vi "CSM - Flush Queue.vi"(8 "Error In":errorcluster caption="error in (no error)", 9 "Option (Low Priority As Default)":enum16{"All", "High Priority", "Low Priority"}(ring)=enum."Low Priority", 11 "CSM Name":string) -> (0 "error out":errorcluster, 1 "#Flushed":cluster{i32, i32}, 3 "CSM Name (Dup)":string)   [LabVIEW 2017, in "Communicable State Machine.lvlib"]
doc: "Clears the LabVIEW queue used in the background for inter-module communication of a CSM module.\n\n> [!NOTE] \n> <b>CSM Priority Queue Design</b>\n>\n> In the background, CSM essentially uses LabVIEW queues to implement inter-module communication. However, CSM uses two separate queues to store messages of different priorities:\n>\n> - <b>Normal Priority Queue:</b> Used for passing asynchronous messages and status broadcasts.\n> - <b>High Priority Message Queue:</b> Used for passing synchronous messages and interrupt broadcasts. Messages in the High Priority Queue are processed first. Messages in the Normal Priority Queue are processed only after the messages in the High Priority Queue have been processed.\n\n\n> [!WARNING] \n> Using this VI is generally not recommended for CSM modules. It is recommended to use code design to avoid message accumulation in modules. Therefore, it is recommended to avoid using this VI to clear background message queues in CSM modules.\n\n-- <b>Controls</b> --\n- <b>CSM Name</b>: CSM module name.\n- <b>Option (Low Priority As Default)</b>: The queue to flush. You can select from the following: All, Low Priority, and High Priority. The default is Low Priority.\n\n-- <b>Indicators</b> --\n- <b>CSM Name (Dup)</b>: A copy of the input CSM module name.\n- <b>#Flushed</b>: Number of elements in the flushed message queue."
uses:
  Communicable State Machine.lvlib
  _Support/CSMQ/_CSMOFGVOPER.ctl
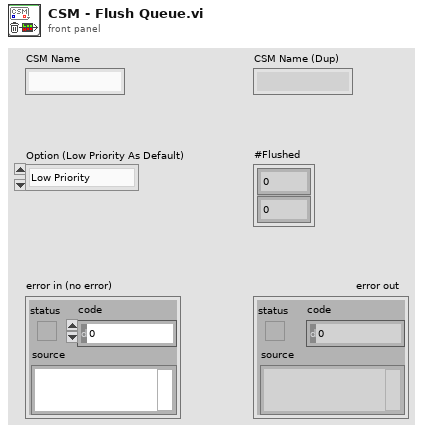
[diagram p1: front panel]
types:
  T1 = typedef "Communicable State Machine.lvlib/_CSMOFGVOPER.ctl" = enum16{"Create If not Exist", "Get By Name", "List", "Check If Name Exists", "Release", "Module Status", "Create Status Event Handler", "Destroy Status Event Handler", "Clear Invalid Objs"}
  T2 = typedef "Communicable State Machine.lvlib/_CSMObj.ctl" = cluster{"info":T3, "Refs":T5}
  T3 = typedef "Communicable State Machine.lvlib/_CSMObj-Info.ctl" = cluster{"Module Name":string, "Requested Name":string, "Group Name":string, "Mode":T4, "Allowed Messages":string[]}
  T4 = typedef "Communicable State Machine.lvlib/_CSM_MODE.ctl" = enum16{"Not Exist", "Stand Alone", "CSM", "Worker", "Worker Agent", "Chain Node", "Chain"}
  T5 = typedef "Communicable State Machine.lvlib/_CSMObj-Refs.ctl" = cluster{"WatchDogQ":refnum<queue>, "CSMDataDVR":refnum<data-value>, "Queue":T6, "GroupDataDVR":refnum<data-value>, "TagMap":refnum<data-value>, "ExitEvent":refnum<user-event>, "NewStateEvent":refnum<user-event>, "StatusEvent":refnum<user-event>, "InterruptEvent":refnum<user-event>}
  T6 = typedef "Communicable State Machine.lvlib/Priority Queue.ctl" = cluster{"HPriorityQ":refnum<queue>, "LowPriorityQ":refnum<queue>}
  T7 = typedef "Communicable State Machine.lvlib/def-Data(LowPRI-Q).ctl" = cluster{"Data":T8, "Notify?":bool}
  T8 = typedef "Communicable State Machine.lvlib/_Cross CSM State Data.ctl" = cluster{"Msg Type":T9, "state":string, "args":string, "source":string, "RespQ":refnum<queue>, "Response For Message":T10, "Target":string}
  T9 = typedef "Communicable State Machine.lvlib/_CSM_MSG_TYPE.ctl" = enum16{"Sync Message(-@)", "Async Message(->)", "Async without Response(->|)", "Async Response", "Broadcast(-><all>)", "Broadcast(-><status>)", "Broadcast(-><interrupt>)", "Append to JKISM States", "Append to JKISM States(High Priority)", "Broadcast(-><state>)"}
  T10 = typedef "Communicable State Machine.lvlib/_CSM_Response Source Message.ctl" = cluster{"‘State":string, "’Arguments":string, "’Error":errorcluster}
  T11 = typedef "Communicable State Machine.lvlib/_CSMObj-ModeData.ctl" = cluster{"CSMDataDVR":refnum<data-value>[], "PriorityQueues":T6[], "Messages of Chain Nodes":cluster{"Module Name":string, "Allowed Messages":string[]}[], "Chain Message Mapping Map":variant, "SharedRegistryRules":string[]}
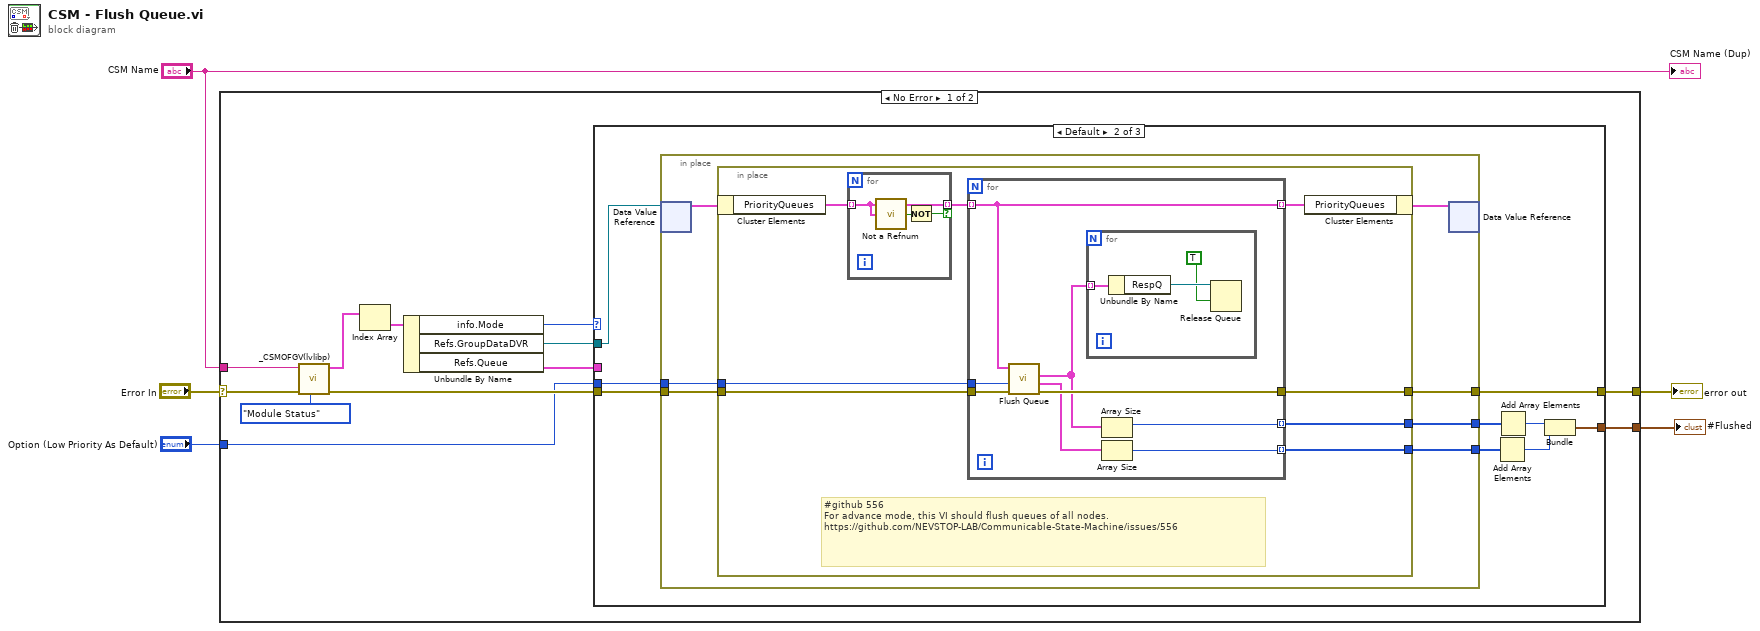
[diagram p0: block diagram]
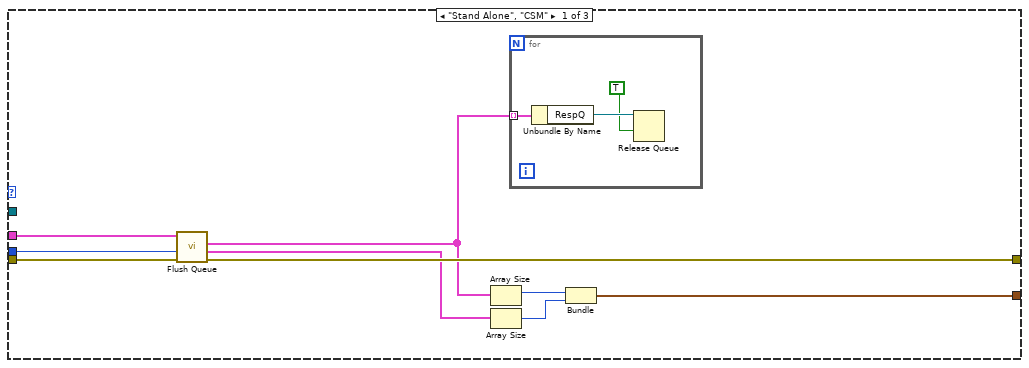
[diagram p2: hidden frame]
diagram:
  n1 = case shown="No Error" "Error In" {
    selector: "Error In" -> [w17 w69]
    tunnel: [w11 w69] -> w4
    tunnel: "CSM Name" -> [w12 _]
    tunnel: "Option (Low Priority As Default)" -> [w9 _]
    tunnel: [w8 _] -> w1
    frame No Error {
      n2 = call "_CSMOFGV(lvlibp).vi"("Operation"=_CSMOFGVOPER."Module Status", "Error In"=w17, "Name (\"\" to Use UUID) In"=w12) -> ("error out"=w10:errorcluster, "Array"=w15:T2[])  [unwired: 6 in, 1 out]
      n3 = Index Array(array=w15) -> (element=w14:T2)  [unwired: 1 in]
      n4 = Unbundle By Name(w14) -> ("info.Mode"=w7:T4, "Refs.GroupDataDVR"=w6:refnum<data-value>, "Refs.Queue"=w13:T6)
      n5 = case shown="Default" w7 {
        tunnel: w13 -> [w26 _ _]
        tunnel: [w25 w38 w68] -> w11
        tunnel: w10 -> [w24 w37 w68]
        tunnel: w9 -> [w23 w36 _]
        tunnel: [w18 w33 _] -> w8
        tunnel: w6 -> [_ w32 _]
        frame "Stand Alone", "CSM" {
          n6 = call "Flush Queue.vi"("error in (no error)"=w24, "Option (Low Priority As Default)"=w23, "Priority Queue In"=w26) -> ("error out"=w25:errorcluster, "Remaining Elements (Low)"=w21:T7[], "Remaining Elements (Hight)"=w22:T8[])  [unwired: 5 in, 1 out]
          n7 = Array Size(array=w22) -> (size(s)=w20:i32)
          n8 = Array Size(array=w21) -> (size(s)=w19:i32)
          n9 = for {
            tunnel: w22 -> [w29] mode=indexing
            n10 = Unbundle By Name(w29) -> ("RespQ"=w28:refnum<queue>)
            n11 = Release Queue(queue=w28, force destroy? (F)=TRUE) -> ()  [unwired: 1 in, 3 out]
          }
          n12 = Bundle(w20, w19) -> (w18:cluster{i32, i32})  [unwired: 1 in]
        }
        frame Default {
          n13 = in-place {
            in-place-border: [w45] -> w38
            in-place-border: w37 -> [w44]
            in-place-border: w36 -> [w43]
            in-place-border: [w42] -> w35
            in-place-border: [w41] -> w34
            n14 = in-place-dvr #1(w32) -> (w40:T11)  [unwired: 1 out]
            n15 = in-place {
              in-place-border: [w53] -> w45
              in-place-border: w44 -> [w52]
              in-place-border: w43 -> [w51]
              in-place-border: [w50] -> w42
              in-place-border: [w49] -> w41
              # "#github 556\nFor advance mode, this VI should flush queues of all nodes.\nhttps://github.com/NEVSTOP-LAB/Communicable-State-Machine/issues/556"
              n16 = in-place-cluster #2(w40) -> ("PriorityQueues"=w47:T6[])
              n17 = for {
                tunnel: w47 -> [w56] mode=indexing
                tunnel: [w56] -> w46 mode=indexing if=w54
                n18 = call "Not a Refnum.vi"("Priority Queue.lvclass"=w56) -> ("NaN/Path/Refnum?"=w55:bool)  [unwired: 4 in]
                n19 = Not(x=w55) -> (.not. x?=w54:bool)
              }
              n20 = for {
                tunnel: w51 -> [w62]
                tunnel: [w59] -> w50 mode=indexing
                tunnel: [w58] -> w49 mode=indexing
                tunnel: w46 -> [w57] mode=indexing
                tunnel: [w57] -> w48 mode=indexing
                tunnel: w52 -> [w63]
                tunnel: [w64] -> w53
                n21 = call "Flush Queue.vi"("error in (no error)"=w63, "Option (Low Priority As Default)"=w62, "Priority Queue In"=w57) -> ("error out"=w64:errorcluster, "Remaining Elements (Low)"=w60:T7[], "Remaining Elements (Hight)"=w61:T8[])  [unwired: 5 in, 1 out]
                n22 = for {
                  tunnel: w61 -> [w67] mode=indexing
                  n23 = Unbundle By Name(w67) -> ("RespQ"=w66:refnum<queue>)
                  n24 = Release Queue(queue=w66, force destroy? (F)=TRUE) -> ()  [unwired: 1 in, 3 out]
                }
                n25 = Array Size(array=w61) -> (size(s)=w59:i32)
                n26 = Array Size(array=w60) -> (size(s)=w58:i32)
              }
              n27 = in-place-cluster #2("PriorityQueues"=w48) -> (w39:T11)
            }
            n28 = in-place-dvr #1(w39) -> ()  [unwired: 2 out]
          }
          n29 = Add Array Elements(numeric array=w34) -> (sum=w30:i32)
          n30 = Add Array Elements(numeric array=w35) -> (sum=w31:i32)
          n31 = Bundle(w31, w30) -> (w33:cluster{i32, i32})  [unwired: 1 in]
        }
        frame "Not Exist" {
        }
      }
    }
    frame Error {
    }
  }
  "error out" <- w4
  "#Flushed" <- w1
  "CSM Name (Dup)" <- "CSM Name"
